vi "edge_detect.vi"() -> ()   [LabVIEW 2019]
uses:
  <vilib>/Platform/TimedLoop/XDataNode/timing_clust.ctl
  <vilib>/Platform/TimedLoop/XDataNode/nitl_modes.ctl
  <vilib>/Platform/TimedLoop/XDataNode/wakeup.ctl
  <vilib>/vision/Measure.llb/Straight Edge Options.ctl
  <vilib>/vision/Measure.llb/Straight Edge Process.ctl
  <vilib>/vision/Measure.llb/Edge Options.ctl
  <vilib>/vision/Measure.llb/Edge Polarity.ctl
  <vilib>/addons/control/pid/pid.llb/PID (DBL).vi
  <vilib>/platform/TimedLoop/XDataNode/XDataNode.xnode
  <vilib>/vision/NI_Vision_Development_Module.lvlib
  <vilib>/Platform/TimedLoop/XDataNode/XDNodeRunTimeDep.lvlib
  <vilib>/addons/control/pid/NI_PID_pid.lvlib
panel:
  out "Waveform Graph 2":waveform(dbl)(graph)={"t0"=timestamp(0 s since 1904-01-01), "dt"=0.1, "Y"=array[1206 elements]} caption="Error [mm]"
  out "PID Send [mm/s]":dbl=1.0 format="%.2f"
  out "Sending Stop":bool=TRUE
  out "Frequency_Send [Hz]":dbl=2.5
  out "dt_Send [ms]":u32=400
  out "concatenated string":string="1.00\r"
  out "error out":errorcluster
  out "Robot Velocity Send [mm/s]":dbl[](graph)=[9.17798733804321, 9.17798733804321, 9.17798733804321, 9.17798733804321, 9.17798733804321, 9.169909177947993, 9.226906974914549, 9.296583231567382, 9.195852826843257, 9.218335621887206, 9.221515865966794, 9.133336371032712, 8.703187100952142, 9.205589135589598, 9.082452465759275, 9.220206353698728, 9.211626497344966, 8.863253717407225, 9.22766377096557, 8.741537103088376, 9.116185161651607, 8.767914421630856, 9.12593847705078, 9.313878997497554, 8.708586713226317, 9.213497229156488, 9.040871199584956, 9.161805507873531, 9.2115924840393, 9.21345471252441, 9.122401093261715, 9.249134670166015, 9.176958435546872, 9.243360911529535, 9.179713513305657, 9.230240278869623, 9.261141367065427, 9.209951342041009, 9.22480665328979, 8.670041134582519, 8.75181762472534, 9.252331920898435, 9.248811543762201, 9.242850711944577, 9.257867586395257, 9.13687375482177, 9.27880277603149, 9.259389681823727, 8.75868831246948, 9.25586080136108, 9.191439600433348, 9.318402767150879, 9.242306499053953, 9.273258607208248, 9.28113268746948, 9.23156679779052, 9.263284205322265, 9.275903141723632, 8.821374834808346, 9.275086822387692, 9.263003595550536, 9.284695581237791, 9.135802335693356, 9.192970199188231, 9.156439908905028, 9.24398165435791, 9.194135154907222, 9.278292576446532, 9.10421247805786, 9.129186747741699, 9.14490939828491, 9.247110878478999, 9.274287509704585, 9.289959140289305, 9.265495070190426, 9.257127796997068, 9.200317073211664, 8.823194546661377, 9.108209041473387, 9.264678750854486, 8.827548249786375, 9.265248473724363, 9.1238806720581, 9.23966196453857, 8.71220062695312, 9.300579794982909, 9.141482557739252, 9.273879350036616, 8.838441010925287, 9.3775093890686, 9.160113345916741, 9.243820091156003, 9.271753518432611, 9.18422027630615, 9.180920985656734, 9.22086110983276, 10.0, 10.0, 10.0, 10.0, 10.0, 10.0, 10.0, 10.0, 10.0, 10.0, 10.0, 10.0, 10.0, 10.0, 10.0, 10.0, 10.0, 10.0, 10.0, 10.0, 10.0, 10.0, 1.0, 1.0, 1.0, 1.0, 1.0, 1.0, 1.0, 1.0, 1.0, 1.0, 1.0, 1.0, 1.0, 1.0, 1.0, 1.0, 1.0, 1.0, 1.0, 1.0, 1.0, 1.0, 1.0, 1.0, 1.0, 1.0, 1.0, 1.0, 1.0, 1.0, 1.0, 1.0, 1.0, 1.0, 1.0, 1.0, 1.0, 1.0, 1.0, 1.0, 1.0, 1.0, 1.0, 1.0, 1.0, 1.0, 1.0, 1.0, 1.0, 1.0, 1.0, 1.0, 1.0, 1.0, 1.0, 1.0, 1.0, 1.0, 1.0, 1.0, 1.0, 1.0, 1.0, 1.0, 1.0, 1.0, 1.0, 1.0, 1.0, 1.0, 1.0, 1.0, 1.0, 1.0, 1.0, 1.0, 1.0, 1.0, 1.0, 1.0, 1.0, 1.0, 1.0, 1.0, 1.0, 1.0, 1.0, 1.0, 1.0, 1.0, 1.0, 1.0, 1.0, 1.0, 1.0, 1.0, 1.0, 1.0, 1.0, 1.0, 1.0, 1.0, 1.0, 1.0, 1.0, 1.0, 1.0, 1.0, 1.0, 1.0, 1.0, 1.0, 1.0, 1.0, 1.0, 1.0, 1.0, 1.0, 1.0, 1.0, 1.0, 1.0, 1.0, 1.0, 1.0, 1.0, 1.0, 1.0, 1.0, 1.0, 1.0, 1.0, 1.0, 1.0, 1.0, 1.0, 1.0, 1.0, 1.0, 1.0, 1.0, 1.0, 1.0, 1.0, 1.0, 1.0, 1.0, 1.0, 1.0, 1.0, 1.0, 1.0, 1.0, 1.0, 1.0, 1.0, 1.0, 1.0, 1.0, 1.0, 1.0, 1.0, 1.0, 1.0, 1.0, 1.0, 1.0, 1.0, 1.0, 1.0, 1.0, 1.0, 1.0, 1.0, 1.0, 1.0, 1.0, 1.0, 1.0, 1.0, 1.0, 1.0, 1.0, 1.0, 1.0, 1.0, 1.0, 1.0, 1.0]
  out "Waveform Graph":waveform(dbl)(graph)={"t0"=timestamp(0 s since 1904-01-01), "dt"=0.1, "Y"=array[1206 elements]} caption="Robot Velocity [mm/s]"
  in  "Stop":bool
  out "dt out (s)":dbl=0.1 format="%.3f"
  out "PID output [mm/s]":dbl=1.0 format="%.2f"
  in  "Reference [mm]":dbl=50.0 format="%.2f"
  in  "PID gains":T1={"proportional gain (Kc)"=20.0, "integral time (Ti, min)"=5.0, "derivative time (Td, min)"=1.0} {"derivative time (Td, min)" format="%.3f"; "integral time (Ti, min)" format="%.3f"; "proportional gain (Kc)" format="%.3f"}
  in  "Robot Velocity Range [mm/s]":cluster{"Max":dbl, "Min":dbl}={"Max"=100.0, "Min"=0.0} {"Min" format="%.2f"; "Max" format="%.2f"}
  out "Frequency_Read [Hz]":dbl=10.0
  out "dt_Read [ms]":u32=100
  in  "[mm/pixel]":dbl=0.278637
  out "Width [mm]":sgl=90.653824
  out "Width [pixel]":sgl=325.3474
  out "?":T2(plugin-control)
  out "Straight Edges":T3(array[cluster])=[{"Point1 (Pixels)"={"X"=203.0107, "Y"=99.0}, "Point2 (Pixels)"={"X"=279.38165, "Y"=470.0}, "Point1 (Real-World)"={"X"=203.0107, "Y"=99.0}, "Point2 (Real-World)"={"X"=279.38165, "Y"=470.0}, "Angle (Pixel)"=11.631944450210185, "Angle (Real-World)"=11.631944450210185, "Score"=133.33333333333331, "Straightness"=0.21897972208745078, "Average SNR (db)"=176.89634617534912, "Calibration Valid"=TRUE}] {"Point2 (Real-World)"."Y" format="%.2f"; "Point2 (Real-World)"."X" format="%.2f"; "Point1 (Real-World)"."Y" format="%.2f"; "Point1 (Real-World)"."X" format="%.2f"; "Point2 (Pixels)"."Y" format="%.2f"; "Point2 (Pixels)"."X" format="%.2f"; "Point1 (Pixels)"."Y" format="%.2f"; "Point1 (Pixels)"."X" format="%.2f"}
  out "Straight Edges 2":T3(array[cluster])=[{"Point1 (Pixels)"={"X"=593.84595, "Y"=99.0}, "Point2 (Pixels)"={"X"=539.2412, "Y"=470.0}, "Point1 (Real-World)"={"X"=593.84595, "Y"=99.0}, "Point2 (Real-World)"={"X"=539.2412, "Y"=470.0}, "Angle (Pixel)"=-8.372825532828088, "Angle (Real-World)"=-8.372825532828088, "Score"=113.72549019607843, "Straightness"=7.89902554927001, "Average SNR (db)"=244.02609279450132, "Calibration Valid"=TRUE}] {"Point2 (Real-World)"."Y" format="%.2f"; "Point2 (Real-World)"."X" format="%.2f"; "Point1 (Real-World)"."Y" format="%.2f"; "Point1 (Real-World)"."X" format="%.2f"; "Point2 (Pixels)"."Y" format="%.2f"; "Point2 (Pixels)"."X" format="%.2f"; "Point1 (Pixels)"."Y" format="%.2f"; "Point1 (Pixels)"."X" format="%.2f"}
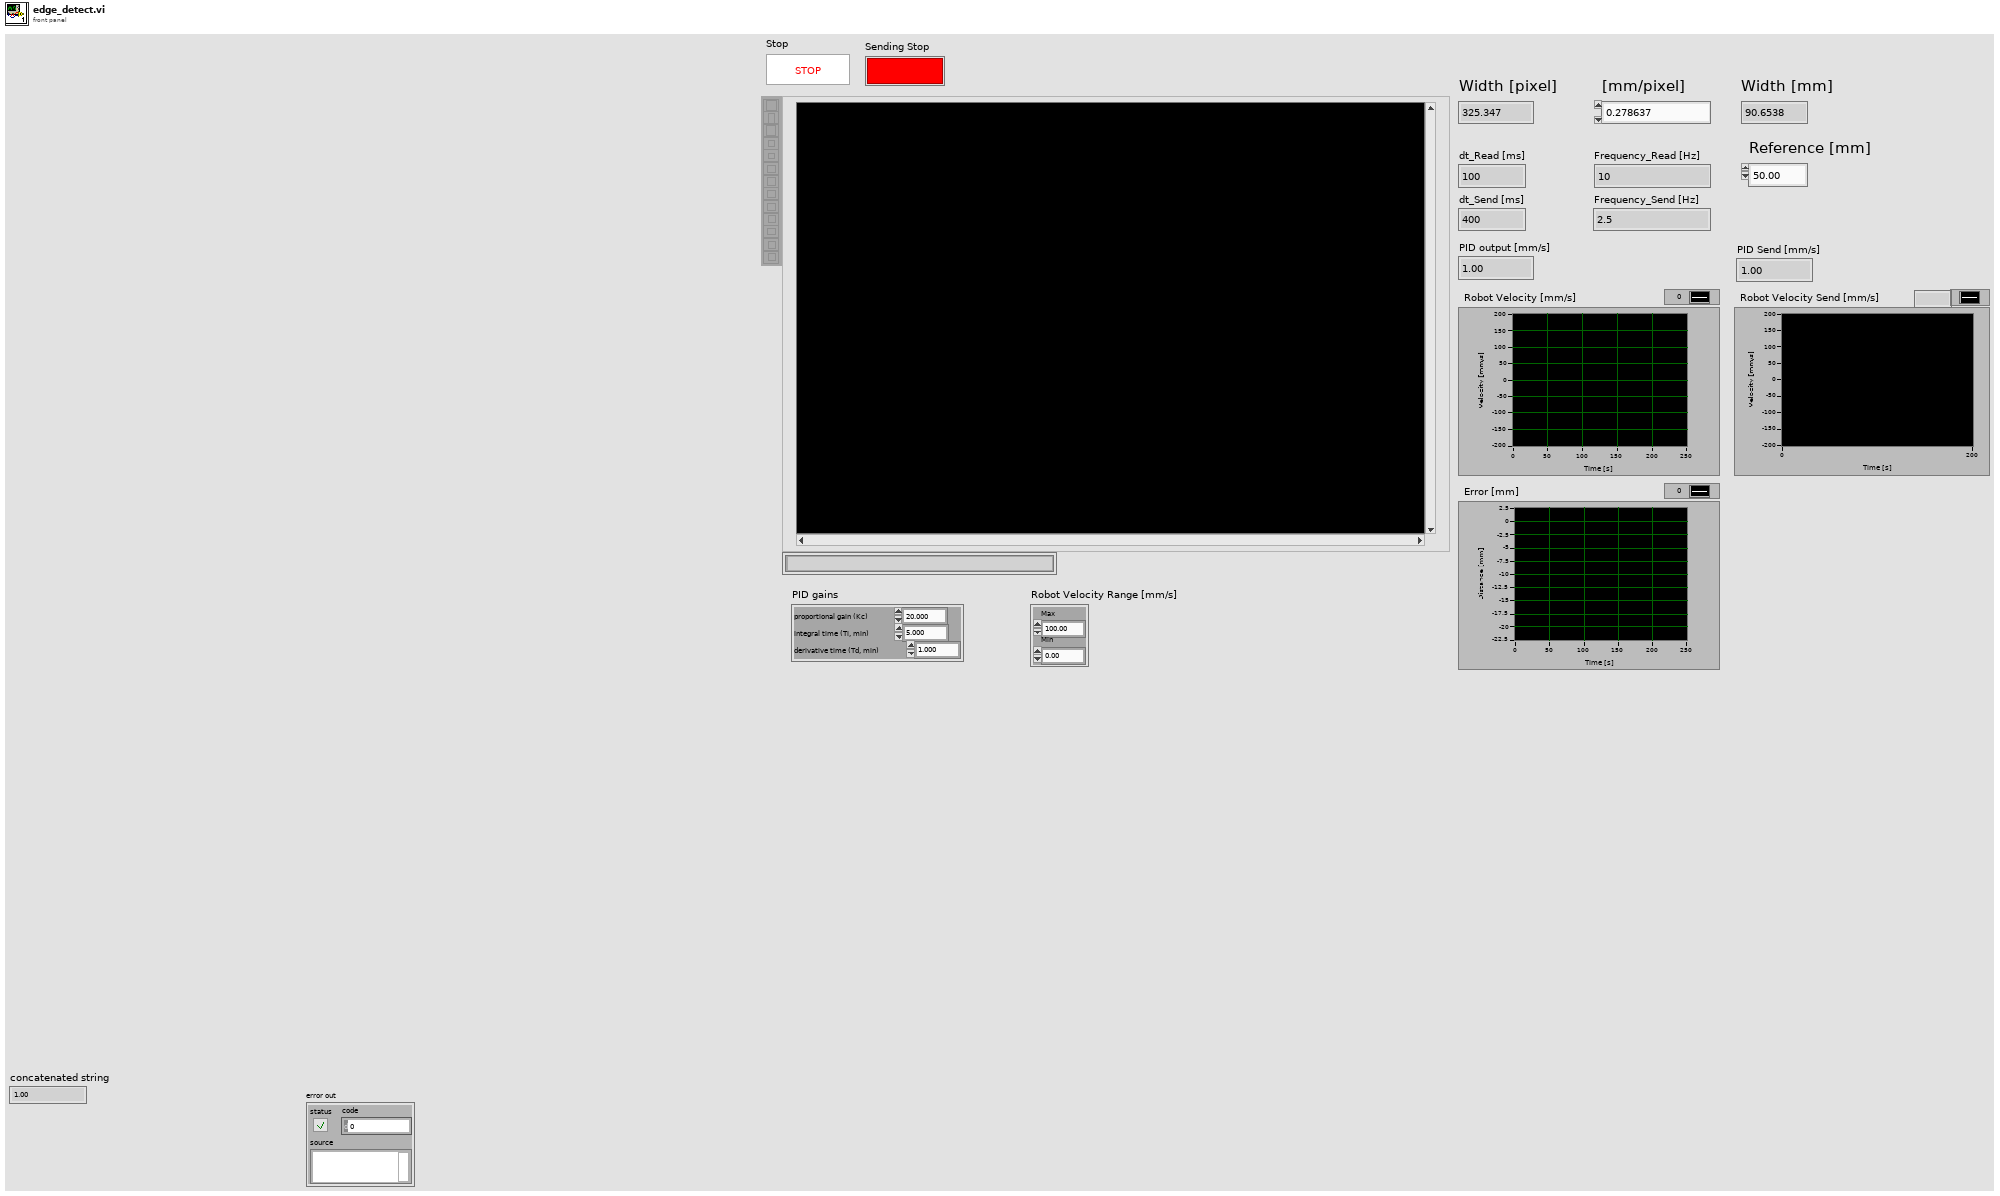
[diagram p1: front panel]
types:
  T1 = cluster{"proportional gain (Kc)":dbl, "integral time (Ti, min)":dbl, "derivative time (Td, min)":dbl}
  T2 = typedef "IMAQ Image.ctl" = refnum<image>
  T3 = cluster{"Point1 (Pixels)":cluster{"X":sgl, "Y":sgl}, "Point2 (Pixels)":cluster{"X":sgl, "Y":sgl}, "Point1 (Real-World)":cluster{"X":sgl, "Y":sgl}, "Point2 (Real-World)":cluster{"X":sgl, "Y":sgl}, "Angle (Pixel)":dbl, "Angle (Real-World)":dbl, "Score":dbl, "Straightness":dbl, "Average SNR (db)":dbl, "Calibration Valid":bool}[]
  T4 = typedef "XDNodeRunTimeDep.lvlib/timing_clust.ctl" = cluster{"Expected End [f-1]":u64, "Actual End [f-1]":u64, "Finished Late? [f-1]":bool, "Expected End [i-1]":u64, "Actual End [i-1]":u64, "Finished Late? [i-1]":bool, "Expected Start [i]":u64, "Actual Start [i]":u64, "Expected Start [f]":u64, "Actual Start [f]":u64, "Source Name":string, "Structure Name":string, "Period":i64, "Deadline":i64, "Offset":i64, "Start":i64, "Priority":i32, "Timeout":i32, "Mode":T5, "Wakeup Reason":T6, "Error":errorcluster, "Source Type":string, "Secondary Source Type":string, "Global End Time":u64, "Global Start Time":u64, "Frame Duration":u64, "Iteration Duration":u64, "Assigned CPU":i32, "I/O Scan Engine Mode":u32}
  T5 = typedef "XDNodeRunTimeDep.lvlib/nitl_modes.ctl" = enum32{"No Change", "Process missed periods, maintain original phase", "Discard missed periods, maintain original phase", "Process missed periods, ignore original phase", "Discard missed periods, ignore original phase"}
  T6 = typedef "XDNodeRunTimeDep.lvlib/wakeup.ctl" = enum32{"Normal", "Aborted", "Asynchronous wakeup", "Timing source error", "Timed loop error", "Timeout"}
  T7 = typedef "Edge Options.ctl" = cluster{"Edge Polarity":T8, "Kernel Size":u32, "Width":u32, "Minimum Edge Strength":sgl, "Interpolation Type":enum32{"Zero Order", "Bilinear", "Quadratic", "Cubic", "Bilinear Fixed"}, "Data Processing Method":enum32{"Average", "Median"}}
  T8 = typedef "Edge Polarity.ctl" = u32
  T9 = cluster{"Search Direction":u32, "Edge Options":T7, "Show Search Area":bool, "Show Search Lines":bool, "Show Edges Found":bool, "Show Result":bool, "Search Area Color":u32, "Search Lines Color":u32, "Edge Locations Color":u32, "Result Color":u32, "Overlay Group Name":string}
  T10 = cluster{"Desired Font (Application)":enum16{"User-specified Font", "Application Font", "System Font", "Dialog Font"}, "[User-specified Font]":cluster{"Font Name":string, "Size":i16, "Strikeout?":bool, "Italic?":bool, "Underline?":bool, "Outline?":bool, "Shadow?":bool, "Bold?":bool, "Rotation Angle":dbl}, "Horizontal Alignment":i16, "Vertical Alignment":i16}
  T11 = typedef "Straight Edge Options.ctl" = cluster{"Number of Lines":i32, "Type":T12, "Min. Score":dbl, "Max. Score":dbl, "Orientation":dbl, "Angle Range":dbl, "Angle Tolerance":dbl, "Step Size":u32, "Min. SNR (db)":dbl, "Min. Points (%)":dbl, "Hough Iterations":i32}
  T12 = typedef "Straight Edge Process.ctl" = enum32{"First Edge Rake", "Best Edge Rake", "Hough Edge Rake", "First Edge Projection", "Best Edge Projection"}
  T13 = cluster{"Global Rectangle":i32[], "Contours":cluster{"Contour Type":u32, "ROI Type":u32, "Points":i32[]}[]}
  T14 = cluster{"Straight Edges[0]":cluster{"Point1 (Pixels)":cluster{"X":sgl, "Y":sgl}, "Point2 (Pixels)":cluster{"X":sgl, "Y":sgl}, "Point1 (Real-World)":cluster{"X":sgl, "Y":sgl}, "Point2 (Real-World)":cluster{"X":sgl, "Y":sgl}, "Angle (Pixel)":dbl, "Angle (Real-World)":dbl, "Score":dbl, "Straightness":dbl, "Average SNR (db)":dbl, "Calibration Valid":bool}, "Straight Edges[1]":cluster{"Point1 (Pixels)":cluster{"X":sgl, "Y":sgl}, "Point2 (Pixels)":cluster{"X":sgl, "Y":sgl}, "Point1 (Real-World)":cluster{"X":sgl, "Y":sgl}, "Point2 (Real-World)":cluster{"X":sgl, "Y":sgl}, "Angle (Pixel)":dbl, "Angle (Real-World)":dbl, "Score":dbl, "Straightness":dbl, "Average SNR (db)":dbl, "Calibration Valid":bool}, "Straight Edges[2]":cluster{"Point1 (Pixels)":cluster{"X":sgl, "Y":sgl}, "Point2 (Pixels)":cluster{"X":sgl, "Y":sgl}, "Point1 (Real-World)":cluster{"X":sgl, "Y":sgl}, "Point2 (Real-World)":cluster{"X":sgl, "Y":sgl}, "Angle (Pixel)":dbl, "Angle (Real-World)":dbl, "Score":dbl, "Straightness":dbl, "Average SNR (db)":dbl, "Calibration Valid":bool}, "Straight Edges[3]":cluster{"Point1 (Pixels)":cluster{"X":sgl, "Y":sgl}, "Point2 (Pixels)":cluster{"X":sgl, "Y":sgl}, "Point1 (Real-World)":cluster{"X":sgl, "Y":sgl}, "Point2 (Real-World)":cluster{"X":sgl, "Y":sgl}, "Angle (Pixel)":dbl, "Angle (Real-World)":dbl, "Score":dbl, "Straightness":dbl, "Average SNR (db)":dbl, "Calibration Valid":bool}, "Straight Edges[4]":cluster{"Point1 (Pixels)":cluster{"X":sgl, "Y":sgl}, "Point2 (Pixels)":cluster{"X":sgl, "Y":sgl}, "Point1 (Real-World)":cluster{"X":sgl, "Y":sgl}, "Point2 (Real-World)":cluster{"X":sgl, "Y":sgl}, "Angle (Pixel)":dbl, "Angle (Real-World)":dbl, "Score":dbl, "Straightness":dbl, "Average SNR (db)":dbl, "Calibration Valid":bool}, "Straight Edges[5]":cluster{"Point1 (Pixels)":cluster{"X":sgl, "Y":sgl}, "Point2 (Pixels)":cluster{"X":sgl, "Y":sgl}, "Point1 (Real-World)":cluster{"X":sgl, "Y":sgl}, "Point2 (Real-World)":cluster{"X":sgl, "Y":sgl}, "Angle (Pixel)":dbl, "Angle (Real-World)":dbl, "Score":dbl, "Straightness":dbl, "Average SNR (db)":dbl, "Calibration Valid":bool}, "Straight Edges[6]":cluster{"Point1 (Pixels)":cluster{"X":sgl, "Y":sgl}, "Point2 (Pixels)":cluster{"X":sgl, "Y":sgl}, "Point1 (Real-World)":cluster{"X":sgl, "Y":sgl}, "Point2 (Real-World)":cluster{"X":sgl, "Y":sgl}, "Angle (Pixel)":dbl, "Angle (Real-World)":dbl, "Score":dbl, "Straightness":dbl, "Average SNR (db)":dbl, "Calibration Valid":bool}, "Straight Edges[7]":cluster{"Point1 (Pixels)":cluster{"X":sgl, "Y":sgl}, "Point2 (Pixels)":cluster{"X":sgl, "Y":sgl}, "Point1 (Real-World)":cluster{"X":sgl, "Y":sgl}, "Point2 (Real-World)":cluster{"X":sgl, "Y":sgl}, "Angle (Pixel)":dbl, "Angle (Real-World)":dbl, "Score":dbl, "Straightness":dbl, "Average SNR (db)":dbl, "Calibration Valid":bool}, "Straight Edges[8]":cluster{"Point1 (Pixels)":cluster{"X":sgl, "Y":sgl}, "Point2 (Pixels)":cluster{"X":sgl, "Y":sgl}, "Point1 (Real-World)":cluster{"X":sgl, "Y":sgl}, "Point2 (Real-World)":cluster{"X":sgl, "Y":sgl}, "Angle (Pixel)":dbl, "Angle (Real-World)":dbl, "Score":dbl, "Straightness":dbl, "Average SNR (db)":dbl, "Calibration Valid":bool}}
  T15 = cluster{"Point1 (Pixels)":cluster{"X":sgl, "Y":sgl}, "Point2 (Pixels)":cluster{"X":sgl, "Y":sgl}, "Point1 (Real-World)":cluster{"X":sgl, "Y":sgl}, "Point2 (Real-World)":cluster{"X":sgl, "Y":sgl}, "Angle (Pixel)":dbl, "Angle (Real-World)":dbl, "Score":dbl, "Straightness":dbl, "Average SNR (db)":dbl, "Calibration Valid":bool}
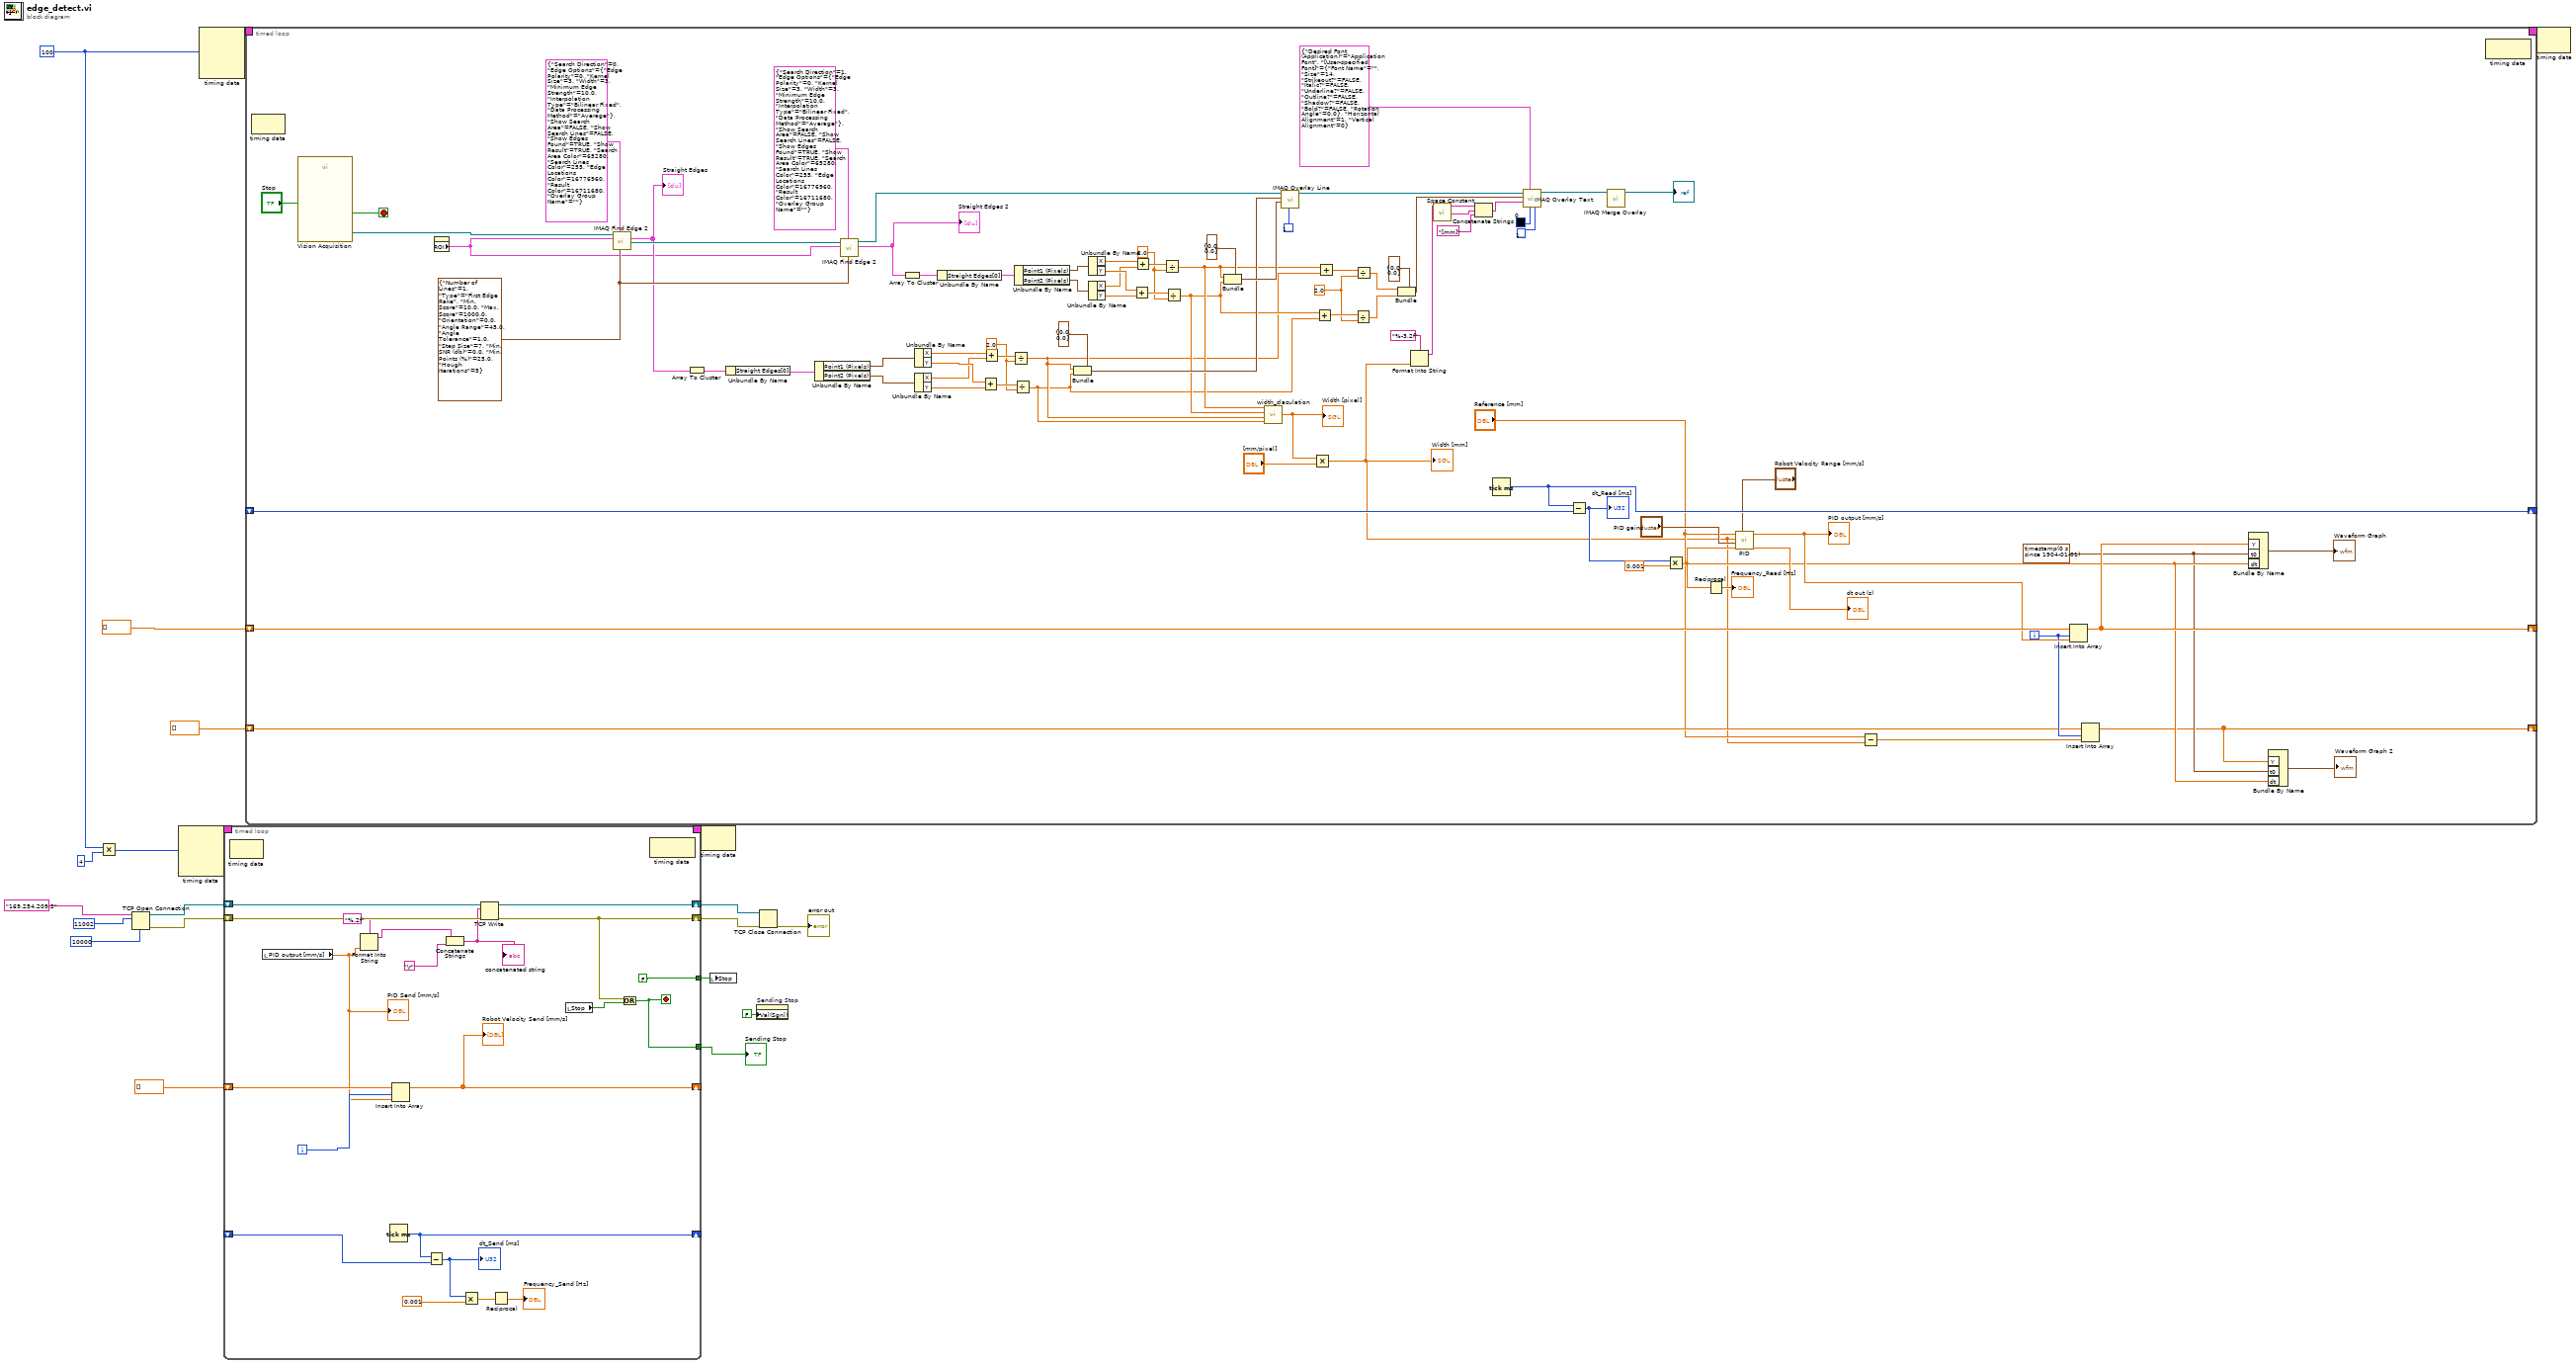
[diagram p0: block diagram]
diagram:
  w6 = i64 100 ("Period")
  n1 = Multiply(x=w6, y=i64 4 ("Period")) -> (x*y=w8:i64)
  n2 = TCP Open Connection(address="169.254.209.2" ("name"), remote port or service name=u16 11002, timeout ms (60000)=10000) -> (connection ID=w14:refnum<k5>, error out=w13:errorcluster)  [unwired: 2 in]
  n3 = node-c288(w8) -> (w18:T4)  [unwired: 3 in]
  n4 = node-c288(w6) -> (w21:T4)  [unwired: 3 in]
  n5 = timed-loop {
    timing: w18 -> [_]
    timing-out: [_] -> w17
    shift-right: [w40] -> w12
    shift-left: w14 -> [w42]
    shift-right: [w29] -> w11
    shift-left: w13 -> [w41]
    shift-right: [w34] -> _
    shift-left: _ -> [w35]
    tunnel: [w28] -> w5
    tunnel: [FALSE ("Stop")] -> w3
    shift-right: [w24] -> _
    shift-left: dbl[] [] ("array") -> [w25]
    i -> [w23]
    stop <- w28 stop-if-true
    n6 = node-c288() -> ()  [unwired: 1 in, 1 out]
    n7 = local read "PID output [mm/s]"() -> (w22:dbl)
    "PID Send [mm/s]" <- w22
    n8 = Format Into String(format string="%.2f", w22) -> (resulting string=w37:string)  [unwired: 2 in, 1 out]
    n9 = Tick Count (ms)() -> (millisecond timer value=w34:u32)
    n10 = Insert Into Array(array=w25, index=w23, new element=w22) -> (w24:dbl[])
    "Robot Velocity Send [mm/s]" <- w24
    n11 = Subtract(x=w34, y=w35) -> (x-y=w26:u32)
    "dt_Send [ms]" <- w26
    n12 = Concatenate Strings(w37, "\r") -> (w38:string)
    "concatenated string" <- w38
    n13 = Multiply(x=w26, y=0.001) -> (x*y=w32:dbl)
    n14 = TCP Write(connection ID=w42, data in=w38, error in (no error)=w41) -> (connection ID out=w40:refnum<k5>, error out=w29:errorcluster)  [unwired: 1 in, 1 out]
    n15 = Reciprocal(x=w32) -> (1/x=→"Frequency_Send [Hz]":dbl)
    n16 = local read "Stop"() -> (w30:bool)
    n17 = Or(x=w29, y=w30) -> (x .or. y?=w28:bool)
    n18 = node-c288() -> ()  [unwired: 1 in, 1 out]
  }
  "Sending Stop" <- w5
  n19 = timed-loop {
    timing: w21 -> [_]
    timing-out: [_] -> w20
    shift-right: [w70] -> _
    shift-left: _ -> [w71]
    shift-right: [w58] -> _
    shift-left: dbl[] [] -> [w62]
    shift-right: [w48] -> _
    shift-left: dbl[] [] -> [w51]
    i -> [w53]
    stop <- w125 stop-if-true
    w49 = timestamp(0 s since 1904-01-01) ("t0")
    w97 = sgl 2.0 ("y")
    w103 = sgl 2.0 ("y")
    w117 = sgl 2.0 ("y")
    w124 = T11 {"Number of Lines"=1, "Type"=enum."First Edge Rake", "Min. Score"=10.0, "Max. Score"=1000.0, "Orientation"=0.0, "Angle Range"=45.0, "Angle Tolerance"=1.0, "Step Size"=7, "Min. SNR (db)"=0.0, "Min. Points (%)"=25.0, "Hough Iterations"=5} ("Line Fit Options")
    n20 = node-c288() -> ()  [unwired: 1 in, 1 out]
    n21 = call "Vision Acquisition"("Stop (F)"="Stop") -> ("Image Out"=w126:T2, "Stopped"=w125:bool)  [unwired: 24 in, 1 out]
    n22 = property class="ImageControl"() -> ("ROI"=w84:T13)  [unwired: 2 in, 2 out]
    n23 = call "IMAQ Find Edge 2"("Line Fit Options"=w124, "Options"=T9 {"Search Direction"=0, "Edge Options"={"Edge Polarity"=0, "Kernel Size"=3, "Width"=3, "Minimum Edge Strength"=10.0, "Interpolation Type"=enum."Bilinear Fixed", "Data Processing Method"=enum."Average"}, "Show Search Area"=FALSE, "Show Search Lines"=FALSE, "Show Edges Found"=TRUE, "Show Result"=TRUE, "Search Area Color"=65280, "Search Lines Color"=255, "Edge Locations Color"=16776960, "Result Color"=16711680, "Overlay Group Name"=""}, "ROI Descriptor"=w84, "Image"=w126) -> ("Straight Edges"=w123:T3, "Image Out"=w127:T2)  [unwired: 4 in, 2 out]
    "Straight Edges" <- w123
    n24 = Array To Cluster(array=w123) -> (cluster=w122:T14)
    n25 = Unbundle By Name(w122) -> ("Straight Edges[0]"=w121:T15)
    n26 = Unbundle By Name(w121) -> ("Point1 (Pixels)"=w116:cluster{"X":sgl, "Y":sgl}, "Point2 (Pixels)"=w120:cluster{"X":sgl, "Y":sgl})
    n27 = call "IMAQ Find Edge 2"("Line Fit Options"=w124, "Options"=T9 {"Search Direction"=1, "Edge Options"={"Edge Polarity"=0, "Kernel Size"=3, "Width"=3, "Minimum Edge Strength"=10.0, "Interpolation Type"=enum."Bilinear Fixed", "Data Processing Method"=enum."Average"}, "Show Search Area"=FALSE, "Show Search Lines"=FALSE, "Show Edges Found"=TRUE, "Show Result"=TRUE, "Search Area Color"=65280, "Search Lines Color"=255, "Edge Locations Color"=16776960, "Result Color"=16711680, "Overlay Group Name"=""}, "ROI Descriptor"=w84, "Image"=w127) -> ("Straight Edges"=w112:T3, "Image Out"=w114:T2)  [unwired: 4 in, 2 out]
    "Straight Edges 2" <- w112
    n28 = Array To Cluster(array=w112) -> (cluster=w111:T14)
    n29 = Unbundle By Name(w116) -> ("X"=w79:sgl, "Y"=w78:sgl)
    n30 = Unbundle By Name(w120) -> ("X"=w77:sgl, "Y"=w76:sgl)
    n31 = Unbundle By Name(w111) -> ("Straight Edges[0]"=w110:T15)
    n32 = Add(x=w78, y=w76) -> (x+y=w118:sgl)
    n33 = Add(x=w79, y=w77) -> (x+y=w119:sgl)
    n34 = Divide(x=w119, y=w117) -> (x/y=w73:sgl)
    n35 = Divide(x=w118, y=w117) -> (x/y=w72:sgl)
    n36 = Unbundle By Name(w110) -> ("Point1 (Pixels)"=w107:cluster{"X":sgl, "Y":sgl}, "Point2 (Pixels)"=w106:cluster{"X":sgl, "Y":sgl})
    n37 = Bundle(cluster=cluster{sgl, sgl} {0.0, 0.0}, w73, w72) -> (w102:cluster{sgl, sgl})
    n38 = Unbundle By Name(w107) -> ("X"=w83:sgl, "Y"=w82:sgl)
    n39 = Unbundle By Name(w106) -> ("X"=w81:sgl, "Y"=w80:sgl)
    n40 = Add(x=w82, y=w80) -> (x+y=w108:sgl)
    n41 = Add(x=w83, y=w81) -> (x+y=w109:sgl)
    n42 = Divide(x=w109, y=w103) -> (x/y=w75:sgl)
    n43 = Divide(x=w108, y=w103) -> (x/y=w74:sgl)
    n44 = Bundle(cluster=cluster{sgl, sgl} {0.0, 0.0}, w75, w74) -> (w105:cluster{sgl, sgl})
    n45 = call "width_claculation.vi"("Y2"=w72, "X2"=w73, "Y1"=w74, "X1"=w75) -> ("width"=w101:dbl)
    "Width [pixel]" <- w101
    n46 = call "IMAQ Overlay Line"("Color"=u32 16777228, "End Point"=w105, "Start Point"=w102, "Image"=w114) -> ("Image Out"=w96:T2)  [unwired: 6 in, 1 out]
    n47 = Multiply(x=w101, y="[mm/pixel]") -> (x*y=w45:dbl)
    "Width [mm]" <- w45
    n48 = Add(x=w74, y=w72) -> (x+y=w98:sgl)
    n49 = Add(x=w75, y=w73) -> (x+y=w99:sgl)
    n50 = Divide(x=w98, y=w97) -> (x/y=w94:sgl)
    n51 = Divide(x=w99, y=w97) -> (x/y=w95:sgl)
    n52 = Bundle(cluster=cluster{sgl, sgl} {0.0, 0.0}, w95, w94) -> (w93:cluster{sgl, sgl})
    n53 = Format Into String(format string="%-3.2f", w45) -> (resulting string=w88:string)  [unwired: 2 in, 1 out]
    n54 = call <vilib>:"Space Constant.vi"() -> ("String"=w85:string)
    n55 = Concatenate Strings(w88, w85, "[mm]" ("element")) -> (w87:string)
    n56 = Tick Count (ms)() -> (millisecond timer value=w70:u32)
    n57 = call "IMAQ Overlay Text"("BG Color (Transparent)"=u32 16777216, "Text Color (black)"=u32 0, "Font, Size & Style"=T10 {"Desired Font (Application)"=enum."Application Font", "[User-specified Font]"={"Font Name"="", "Size"=14, "Strikeout?"=FALSE, "Italic?"=FALSE, "Underline?"=FALSE, "Outline?"=FALSE, "Shadow?"=FALSE, "Bold?"=FALSE, "Rotation Angle"=0.0}, "Horizontal Alignment"=1, "Vertical Alignment"=0}, "String"=w87, "Origin"=w93, "Image"=w96) -> ("Image Out"=w54:T2)  [unwired: 4 in, 1 out]
    n58 = Subtract(x=w70, y=w71) -> (x-y=w57:u32)
    "dt_Read [ms]" <- w57
    n59 = call "IMAQ Merge Overlay"("Image Src"=w54) -> ("Image Dst Out"=→"?":T2)  [unwired: 9 in, 1 out]
    n60 = Multiply(x=w57, y=0.001) -> (x*y=w50:dbl)
    n61 = Reciprocal(x=w50) -> (1/x=→"Frequency_Read [Hz]":dbl)
    n62 = call-poly <vilib>:"PID.vi"("output range"="Robot Velocity Range [mm/s]", "dt (s)"=w50, "PID gains"="PID gains", "process variable"=w45, "setpoint"="Reference [mm]") -> ("dt out (s)"=→"dt out (s)":dbl, "output"=w56:dbl)  [unwired: 5 in]
    "PID output [mm/s]" <- w56
    n63 = Subtract(x="Reference [mm]", y=w45) -> (x-y=w52:dbl)
    n64 = Insert Into Array(array=w62, index=w53, new element=w56) -> (w58:dbl[])
    n65 = Insert Into Array(array=w51, index=w53, new element=w52) -> (w48:dbl[])
    n66 = Bundle By Name("Y"=w58, "t0"=w49, "dt"=w50) -> (→"Waveform Graph":waveform(dbl))  [unwired: 1 in]
    n67 = Bundle By Name("Y"=w48, "t0"=w49, "dt"=w50) -> (→"Waveform Graph 2":waveform(dbl))  [unwired: 1 in]
    n68 = node-c288() -> ()  [unwired: 1 in, 1 out]
  }
  n69 = node-c288(w17) -> ()  [unwired: 1 out]
  n70 = local write "Stop"(w3) -> ()
  n71 = property on="Sending Stop" class="Bool (strict)"("Val(Sgnl)"=FALSE ("Value (Signaling)")) -> ()  [unwired: 2 in, 2 out]
  n72 = TCP Close Connection(connection ID=w12, error in (no error)=w11) -> (error out=→"error out":errorcluster)  [unwired: 1 in, 1 out]
  n73 = node-c288(w20) -> ()  [unwired: 1 out]
